vi "SeCrTs-RD Queue Data log module.vi"(8 "error in":errorcluster) -> (0 "error out":errorcluster)   [LabVIEW 2022 SP3]
uses:
  Control/SeCrTs-Datalog enumRD.ctl
  Globals/SeCrTs-RD globals.vi
panel:
  out "x":u32
  out "x-y":dbl
  out "Restart":bool
  out "Log health":bool=TRUE
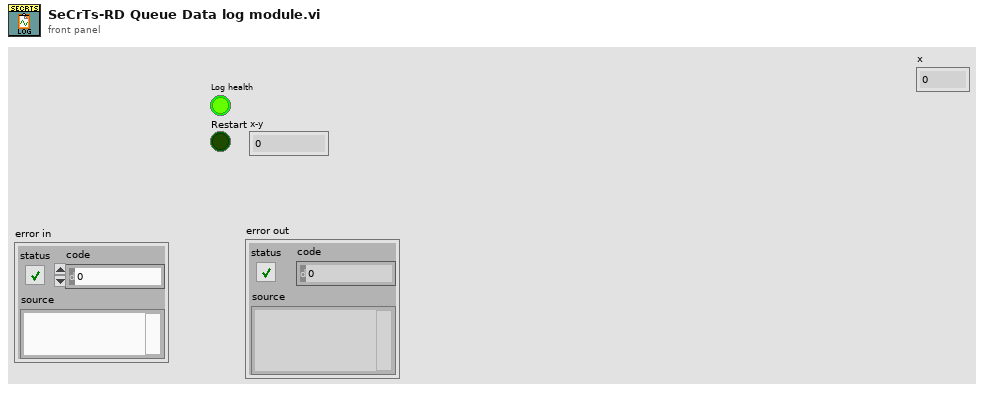
[diagram p1: front panel]
types:
  T1 = cluster{"Log In Progress?":bool, "Log Start Time":timestamp, "Analog Queues":refnum<queue>[], "Digital Queues":refnum<queue>[], "tdms file ref":refnum<k34>}
  T2 = typedef "SeCrTs-Datalog enumRD.ctl" = enum16{"Initialize", "Poll", "Create file", "log Analog", "log Digital", "Flush Queues", "Close file", "Error", "Exit"}
  T3 = enum16{"open", "open or create", "create or replace", "create", "open (read-only)"}
  T4 = cluster{"Datalog path":path, "Configuration path":path, "Signal list path":path, "Sub vi's":path, "Authentication":path}
  T5 = cluster{"analog names":cluster{"AI_C_Data":string[], "AI_V_Data":string[], "AO_Data":string[], "DO_Data":string[], "ACC_Data":string[], "TC Data":string[], "Drive_A_C":string[], "Drive_A_D":string[], "Drive_L_C":string[], "Drive_L_D":string[]}, "Di names":string[]}
  T6 = cluster{"AI_C_Data":string[], "AI_V_Data":string[], "AO_Data":string[], "DO_Data":string[], "ACC_Data":string[], "TC Data":string[], "Drive_A_C":string[], "Drive_A_D":string[], "Drive_L_C":string[], "Drive_L_D":string[]}
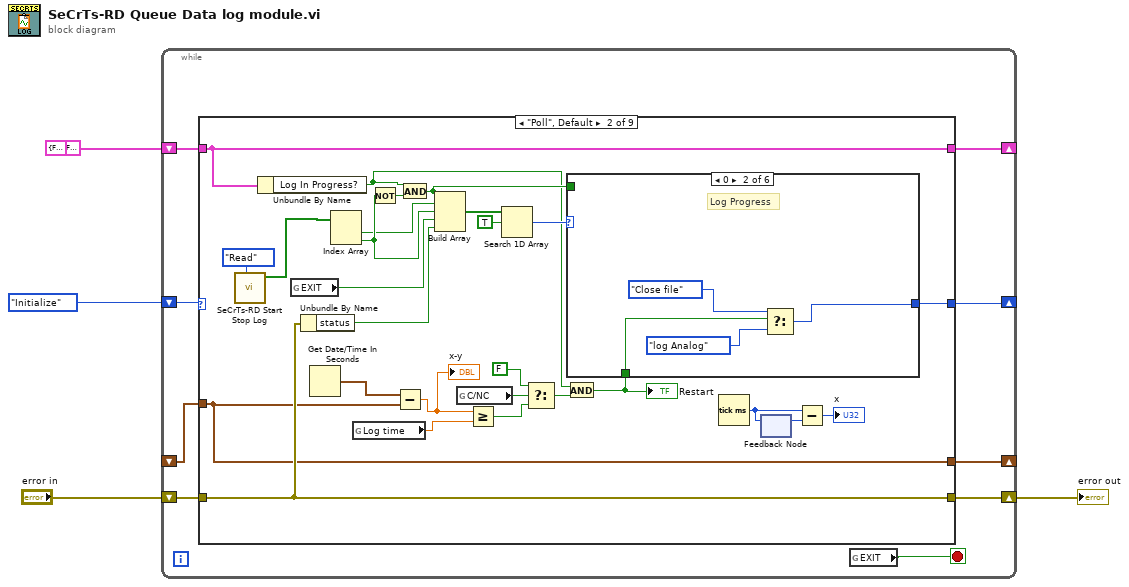
[diagram p0: block diagram]
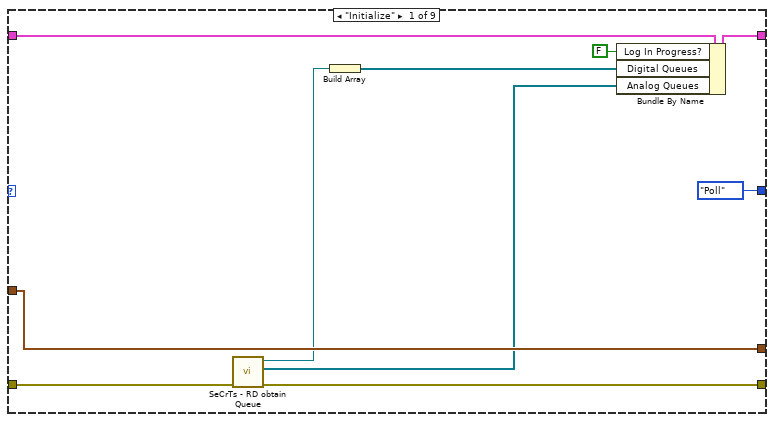
[diagram p2: hidden frame]
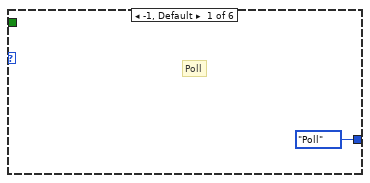
[diagram p3: hidden frame]
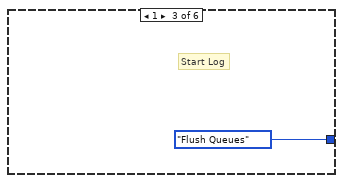
[diagram p4: hidden frame]
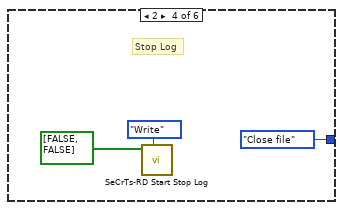
[diagram p5: hidden frame]
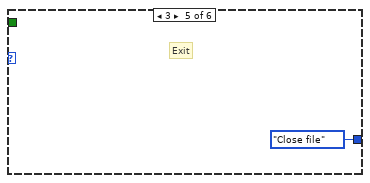
[diagram p6: hidden frame]
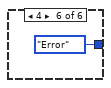
[diagram p7: hidden frame]
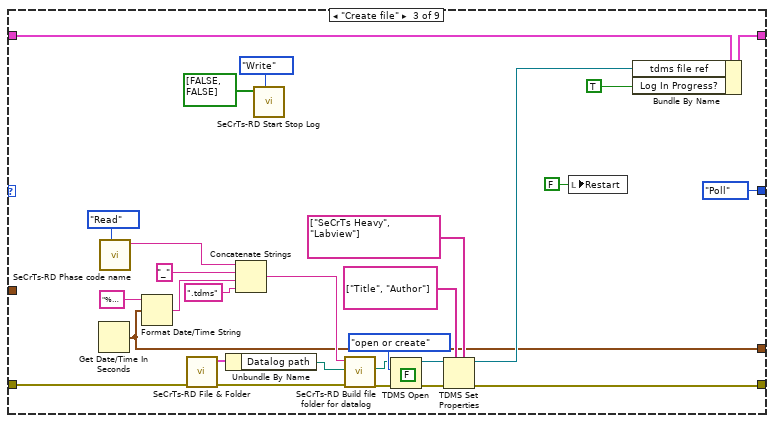
[diagram p8: hidden frame]
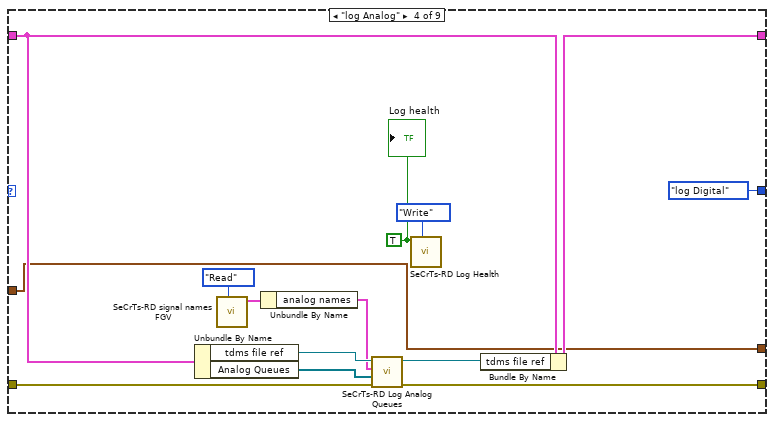
[diagram p9: hidden frame]
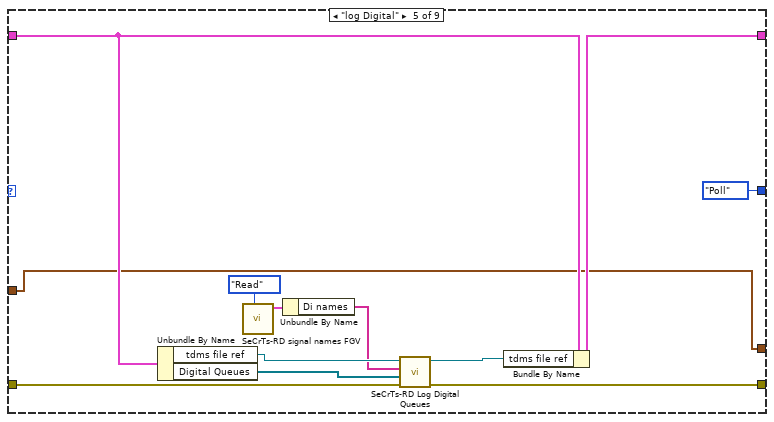
[diagram p10: hidden frame]
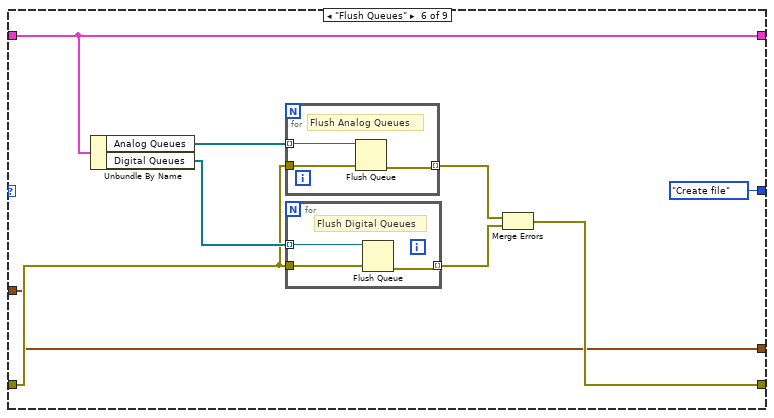
[diagram p11: hidden frame]
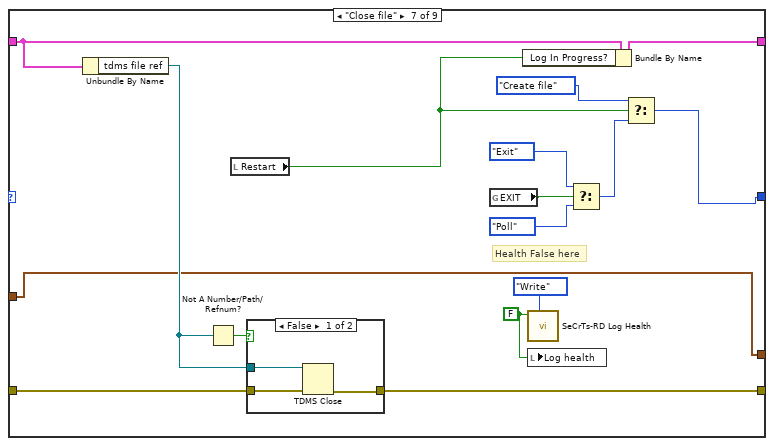
[diagram p12: hidden frame]
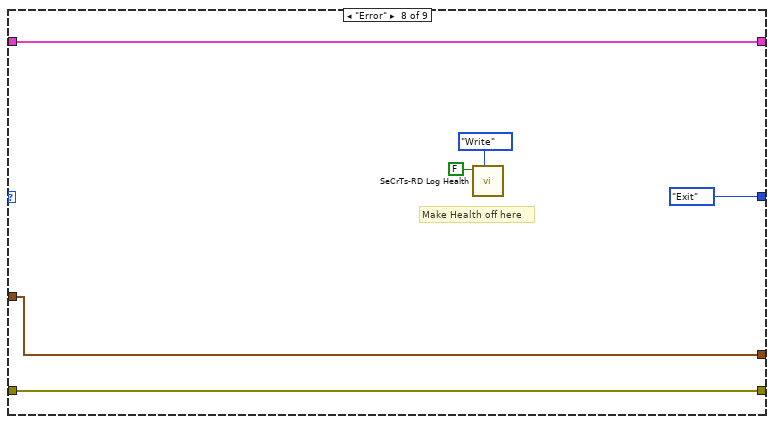
[diagram p14: hidden frame]
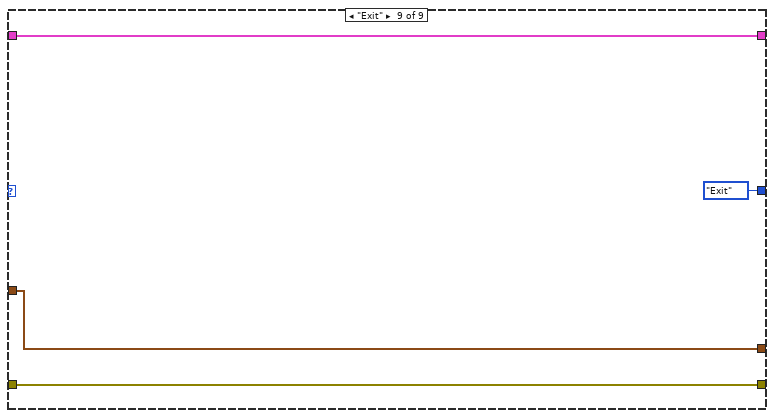
[diagram p15: hidden frame]
diagram:
  (unwired) T1 {"Log In Progress?"=FALSE, "Log Start Time"=timestamp(0 s since 1904-01-01), "Analog Queues"=[], "Digital Queues"=[], "tdms file ref"=refnum}
  n1 = while {
    shift-right: [w8] -> _
    shift-left: SeCrTs-Datalog_enumRD."Initialize" -> [w13]
    shift-right: [w10] -> _
    shift-left: T1 {"Log In Progress?"=FALSE, "Log Start Time"=timestamp(0 s since 1904-01-01), "Analog Queues"=[], "Digital Queues"=[], "tdms file ref"=refnum} -> [w11]
    shift-right: [w9] -> w1
    shift-left: "error in" -> [w12]
    shift-right: [w5] -> _
    shift-left: _ -> [w6]
    stop <- w7 stop-if-true
    n2 = case shown="\"Poll\", Default" w13 {
      tunnel: w12 -> [w18 w44 w84 w100 w114 w120 w142 w154 w159]
      tunnel: w11 -> [w23 w50 w73 w102 w112 w123 w143 w156 w160]
      tunnel: [w22 w50 w72 w97 w109 w123 w144 w156 w160] -> w10
      tunnel: [w17 w44 w69 w99 w113 w117 w141 w154 w159] -> w9
      tunnel: [SeCrTs-Datalog_enumRD."Poll" w45 SeCrTs-Datalog_enumRD."Poll" SeCrTs-Datalog_enumRD."log Digital" SeCrTs-Datalog_enumRD."Poll" SeCrTs-Datalog_enumRD."Create file" w131 SeCrTs-Datalog_enumRD."Exit" SeCrTs-Datalog_enumRD."Exit"] -> w8
      tunnel: w6 -> [w19 w34 _ w90 w104 w116 w135 w151 w157]
      tunnel: [w19 w34 w63 w90 w104 w116 w135 w151 w157] -> w5
      frame "Initialize" {
        n3 = call "SeCrTs - RD obtain Queue.vi"("error in"=w18) -> ("error out"=w17:errorcluster, "Analog Queue"=w14:refnum<queue>[], "DI Data Queue"=w16:refnum<queue>)  [unwired: 8 in]
        n4 = Build Array(w16) -> (w15:refnum<queue>[])
        n5 = Bundle By Name(cluster=w23, "Log In Progress?"=FALSE, "Digital Queues"=w15, "Analog Queues"=w14) -> (w22:T1)
      }
      frame "Poll", Default {
        n6 = call "SeCrTs-RD Start Stop Log.vi"("Enum"=enum16{"Read", "Write"}."Read") -> ("Start Stop log R"=w30:bool[])  [unwired: 9 in, 1 out]
        n7 = Unbundle By Name(w50) -> ("Log In Progress?"=w25:bool)
        n8 = global read "SeCrTs-RD globals.vi" "EXIT"() -> (w40:bool)
        n9 = Unbundle By Name(w44) -> ("status"=w49:bool)
        n10 = Get Date/Time In Seconds() -> (seconds since 1Jan1904=w36:timestamp)
        n11 = Index Array(array=w30) -> (element #1=w41:bool, element #2=w42:bool)  [unwired: 2 in]
        n12 = global read "SeCrTs-RD globals.vi" "Log time"() -> (w29:dbl)
        n13 = Not(x=w42) -> (.not. x?=w43:bool)
        n14 = Subtract(x=w36, y=w34) -> (x-y=w37:dbl)
        "x-y" <- w37
        n15 = And(x=w25, y=w43) -> (x .and. y?=w38:bool)
        n16 = Build Array(w38, w41, w42, w40, w49) -> (w48:bool[])
        n17 = global read "SeCrTs-RD globals.vi" "C/NC"() -> (w28:bool)
        n18 = Greater Or Equal?(x=w37, y=w29) -> (x >= y?=w27:bool)
        n19 = Search 1D Array(1D array=w48, element=TRUE) -> (index of element=w46:i32)  [unwired: 1 in]
        n20 = Select(t=FALSE, s=w28, f=w27) -> (s? t:f=w24:bool)
        n21 = And(x=w25, y=w24) -> (x .and. y?=w35:bool)
        "Restart" <- w35
        n22 = case shown="0" w46 {
          tunnel: [SeCrTs-Datalog_enumRD."Poll" w52 SeCrTs-Datalog_enumRD."Flush Queues" SeCrTs-Datalog_enumRD."Close file" SeCrTs-Datalog_enumRD."Close file" SeCrTs-Datalog_enumRD."Error"] -> w45
          tunnel: w38 -> [_ _ _ _ _ _]
          tunnel: w35 -> [_ w55 _ _ _ _]
          frame -1, Default {
            # "Poll"
          }
          frame 0 {
            # "Log Progress"
            n23 = Select(t=SeCrTs-Datalog_enumRD."Close file", s=w55, f=SeCrTs-Datalog_enumRD."log Analog") -> (s? t:f=w52:T2)
          }
          frame 1 {
            # "Start Log"
          }
          frame 2 {
            # "Stop Log"
            n24 = call "SeCrTs-RD Start Stop Log.vi"("Enum"=enum16{"Read", "Write"}."Write", "Start Stop log"=bool[] [FALSE, FALSE]) -> ()  [unwired: 8 in, 2 out]
          }
          frame 3 {
            # "Exit"
          }
          frame 4 {
          }
        }
        n25 = Tick Count (ms)() -> (millisecond timer value=w32:u32)
        n26 = feedback #1() -> (w33:u32)  [unwired: 1 in]
        n27 = feedback-in #1(w32) -> ()
        n28 = Subtract(x=w32, y=w33) -> (x-y=→"x":u32)
      }
      frame "Create file" {
        (unwired) FALSE ("disable buffering? (T)")
        n29 = Get Date/Time In Seconds() -> (seconds since 1Jan1904=w63:timestamp)
        n30 = call "SeCrTs-RD Phase code name.vi"("Enum"=enum16{"Read", "Write"}."Read") -> ("Phase codeR"=w64:string)  [unwired: 9 in, 1 out]
        n31 = Format Date/Time String(time format string (%c)="%Y_%b_%d_%Hh_%Mm_%Ssec", seconds (now)=w63) -> (date/time string=w89:string)  [unwired: 1 in]
        n32 = call "SeCrTs-RD File & Folder.vi"("error in (no error)"=w84) -> ("error out"=w83:errorcluster, "File Output"=w82:T4)  [unwired: 9 in]
        n33 = Unbundle By Name(w82) -> ("Datalog path"=w81:path)
        n34 = Concatenate Strings(w64, "_" ("string"), w89, ".tdms" ("string")) -> (w85:string)
        n35 = call "SeCrTs-RD Start Stop Log.vi"("Enum"=enum16{"Read", "Write"}."Write", "Start Stop log"=bool[] [FALSE, FALSE]) -> ()  [unwired: 8 in, 2 out]
        n36 = call "SeCrTs-RD Build file folder for datalog.vi"("error in (no error)"=w83, "Base Path"=w81, "File Name"=w85) -> ("error out"=w75:errorcluster, "Result File path"=w74:path)  [unwired: 6 in, 1 out]
        n37 = TDMS Open(8:w75, 10:T3."open or create" ("operation (0:open)"), 11:w74) -> (0:w79:errorcluster, 3:w78:refnum<k34>)  [unwired: 4 in]
        n38 = TDMS Set Properties(5:string[] ["SeCrTs Heavy", "Labview"] ("property names"), 7:string[] ["Title", "Author"] ("property names"), 8:w79, 11:w78) -> (0:w69:errorcluster, 3:w71:refnum<k34>)  [unwired: 4 out]
        n39 = local write "Restart"(FALSE ("Restart")) -> ()
        n40 = Bundle By Name(cluster=w73, "tdms file ref"=w71, "Log In Progress?"=TRUE) -> (w72:T1)
      }
      frame "log Analog" {
        w94 = TRUE ("Log health")
        n41 = Unbundle By Name(w102) -> ("tdms file ref"=w98:refnum<k34>, "Analog Queues"=w101:refnum<queue>[])
        n42 = call "SeCrTs-RD signal names FGV.vi"("Enum"=enum16{"Read", "Write"}."Read") -> ("Signal names R"=w92:T5)  [unwired: 9 in, 1 out]
        n43 = Unbundle By Name(w92) -> ("analog names"=w91:T6)
        n44 = call "SeCrTs-RD Log Analog Queues.vi"("error in"=w100, "Analog queues"=w101, "Channel names"=w91, "tdms file in"=w98) -> ("error out"=w99:errorcluster, "tdms ref out"=w96:refnum<k34>)  [unwired: 6 in]
        n45 = call "SeCrTs-RD Log Health.vi"("Enum"=enum16{"Read", "Write"}."Write", "Log health"=w94) -> ()  [unwired: 8 in, 2 out]
        n46 = Bundle By Name(cluster=w102, "tdms file ref"=w96) -> (w97:T1)
        "Log health" <- w94
      }
      frame "log Digital" {
        n47 = Unbundle By Name(w112) -> ("tdms file ref"=w111:refnum<k34>, "Digital Queues"=w110:refnum<queue>[])
        n48 = call "SeCrTs-RD signal names FGV.vi"("Enum"=enum16{"Read", "Write"}."Read") -> ("Signal names R"=w106:T5)  [unwired: 9 in, 1 out]
        n49 = Unbundle By Name(w106) -> ("Di names"=w105:string[])
        n50 = call "SeCrTs-RD Log Digital Queues.vi"("error in"=w114, "DI_queue"=w110, "DI Names"=w105, "tdms file in"=w111) -> ("error out"=w113:errorcluster, "tdms file out"=w108:refnum<k34>)  [unwired: 6 in]
        n51 = Bundle By Name(cluster=w112, "tdms file ref"=w108) -> (w109:T1)
      }
      frame "Flush Queues" {
        n52 = Unbundle By Name(w123) -> ("Analog Queues"=w122:refnum<queue>[], "Digital Queues"=w121:refnum<queue>[])
        n53 = for {
          tunnel: w122 -> [w130] mode=indexing
          tunnel: w120 -> [w129]
          tunnel: [w128] -> w119 mode=indexing
          # "Flush Analog Queues"
          n54 = Flush Queue(queue=w130, error in (no error)=w129) -> (error out=w128:errorcluster)  [unwired: 2 out]
        }
        n55 = for {
          tunnel: w121 -> [w127] mode=indexing
          tunnel: w120 -> [w126]
          tunnel: [w125] -> w118 mode=indexing
          # "Flush Digital Queues"
          n56 = Flush Queue(queue=w127, error in (no error)=w126) -> (error out=w125:errorcluster)  [unwired: 2 out]
        }
        n57 = Merge Errors(w119, w118) -> (w117:errorcluster)
      }
      frame "Close file" {
        w136 = FALSE ("Log health")
        # "Health False here"
        n58 = Unbundle By Name(w143) -> ("tdms file ref"=w139:refnum<k34>)
        n59 = Not A Number/Path/Refnum?(number/path/refnum=w139) -> (NaN/Path/Refnum?=w140:bool)
        n60 = local read "Restart"() -> (w134:bool)
        n61 = case shown="False" w140 {
          tunnel: w142 -> [w149 w150]
          tunnel: [w148 w150] -> w141
          tunnel: w139 -> [w147 _]
          frame False {
            n62 = TDMS Close(8:w149, 11:w147) -> (0:w148:errorcluster)  [unwired: 1 out]
          }
          frame True {
          }
        }
        n63 = global read "SeCrTs-RD globals.vi" "EXIT"() -> (w137:bool)
        n64 = Bundle By Name(cluster=w143, "Log In Progress?"=w134) -> (w144:T1)
        n65 = call "SeCrTs-RD Log Health.vi"("Enum"=enum16{"Read", "Write"}."Write", "Log health"=w136) -> ()  [unwired: 8 in, 2 out]
        n66 = local write "Log health"(w136) -> ()
        n67 = Select(t=SeCrTs-Datalog_enumRD."Exit", s=w137, f=SeCrTs-Datalog_enumRD."Poll") -> (s? t:f=w132:T2)
        n68 = Select(t=SeCrTs-Datalog_enumRD."Create file", s=w134, f=w132) -> (s? t:f=w131:T2)
      }
      frame "Error" {
        # "Make Health off here"
        n69 = call "SeCrTs-RD Log Health.vi"("Enum"=enum16{"Read", "Write"}."Write", "Log health"=FALSE) -> ()  [unwired: 8 in, 2 out]
      }
      frame "Exit" {
      }
    }
    n70 = global read "SeCrTs-RD globals.vi" "EXIT"() -> (w7:bool)
  }
  "error out" <- w1
